vi "_crosstalk_mkpk.vi"(0 "Bias_LO_equip":T4={"Node address"=19, "CAN Interface"="CAN0", "Cartridge band"=10, "Slave Node in"={"Address"=19, "Serial Number"=[16, -88, -112, 75, 1, 8, 0, 24]}, "ObjHandle out"=93192256, "POL"=0, "sb"=1, "GPIB_SM (SIS S,V)"="24", "GPIB_DMM (SIS I)"="22", "GPIB_SM (MAG I) "="25", "GPIB_SG(LO)"="19", "GPIB_PW (PAMP) "="6", "GPIB_TMP1(8ch)"="12", "GPIB_TMP2(2ch)  "="13", "WCA_avg"=10, "Rsen"=10.0, "BiasModule"=1, "LOModule "=2, "WCA_LO_FREQ_SET"={"YTO Low freq. [GHz]"=14.66, "YTO High freq. [GHz]"=17.5, "Kvco"=1, "Lock Pol."=0, "SET LO FREQ"=88.77778, "Multiplier"=6.0, "YTO (HEX)"=197, "YTO ( FREQ)"=14.796625, "NULL PLL INTEGRATOR"=FALSE}, "Res for"=0} {"Res for" items=["none", "series res", "parallel res"]; "WCA_LO_FREQ_SET"."YTO ( FREQ)" min=25 max=150 step=0.0001 format="%.3f"; "WCA_LO_FREQ_SET"."Multiplier" min=3 max=6 step=3; "WCA_LO_FREQ_SET"."SET LO FREQ" min=25 max=150 step=0.0001 format="%.3f"; "WCA_LO_FREQ_SET"."Lock Pol." items=["Lower", "Upper"]; "WCA_LO_FREQ_SET"."Kvco" items=["7.5MHz/V", "15MHz/V"]; "WCA_LO_FREQ_SET"."YTO High freq. [GHz]" format="%.3f"; "WCA_LO_FREQ_SET"."YTO Low freq. [GHz]" format="%.3f"; "LOModule" items=["Manual Gunn+PAMP"=0, "PLL GUNN+PAMP"=5, "B10Lab LO"=1, "WCA LO"=2, ""=3, "YIG発信器"=4, "none"=99]; "BiasModule" items=["B10Lab Bias"=0, "WCA BiasModule"=1, "none"=99]; "Slave Node in"."Serial Number" format="%.0x"; "Slave Node in"."Address" format="%.0x"; "Cartridge band" max=10 step=1; "Node address" format="%.0x"}, 1 "Control":T8={"GPIB_ATT"="28", "6501Dev#"=1, "GPIB_SP"="18", "GPIB_PM"="13", "GPIB_DSA"="11", "GPIB_DMM (TPD)"="23", "GPIB_MPI"="COM9", "mortor設定"=[{"Axis"=0, "ID"=0, "HIspeed"=200.0, "LOspeed"=100.0, "ACCEL(ms)"=100.0, "Sratio"=50.0, "フリーラン\n"=FALSE, "文字列"="DSB HOT/COLD"}, {"Axis"=1, "ID"=0, "HIspeed"=4.0, "LOspeed"=4.0, "ACCEL(ms)"=100.0, "Sratio"=50.0, "フリーラン\n"=TRUE, "文字列"="SubMM Att"}, {"Axis"=0, "ID"=0, "HIspeed"=200.0, "LOspeed"=100.0, "ACCEL(ms)"=100.0, "Sratio"=50.0, "フリーラン\n"=FALSE, "文字列"="MPI Port1"}, {"Axis"=1, "ID"=0, "HIspeed"=200.0, "LOspeed"=100.0, "ACCEL(ms)"=100.0, "Sratio"=50.0, "フリーラン\n"=FALSE, "文字列"="MPI Port2"}, {"Axis"=1, "ID"=0, "HIspeed"=200.0, "LOspeed"=100.0, "ACCEL(ms)"=100.0, "Sratio"=50.0, "フリーラン\n"=TRUE, "文字列"="gainComp"}], "DATAパス"=path "C:/Documents and Settings/band10/デスクトップ/data/cartridge/CCA03/CCA-03-13/110831_etc", "mixer param file "=path "Z:/band10/Labview_ALMA/MIX95/test", "comment"="xttest", "ColdCarts"="003601", "Th"=299.0, "Tc"=77.0, "Set_SIS_volt"=2.1, "Offset"=0.0, "control"=0, "FreqLO"=799.0, "Set_Mag_Cur"=13.664233576642335, "MPI offset(mm)"=23.152, "HOT/COLD"=0} {"HOT/COLD" items=["DSB", "SBR (Cart.)", "GainComp", "SBR (MIX)"]; "control" items=["CLOSE LOOP", "OPEN LOOP", "Not Control"]}, 2 "CrossTalk_mkpk":T7={"save"=TRUE, "file_name"="xtk_799.00_120_xttest.csv", "IF start"=4.0, "IF stop"=12.0, "IF step"=1.0}, 3 "PAV配列":cluster{"VD":dbl, "VG ":dbl, "文字列":string}[](array[cluster])=[{"VD"=0.0, "VG "=-0.04, "文字列"="WCA P0"}, {"VD"=0.0, "VG "=-0.04, "文字列"="WCA P1"}, {"VD"=1.75, "VG "=2.1, "文字列"="B10 PAMP"}] {"VG" min=-1.0 max=4.0; "VD" min=0.0 max=2.5}, 4 "_LO_P_OPT":T3={"範囲配列"=[{"Start"=1.0, "Stop"=3.5, "Step"=0.01, "ｂｙ"="NEL VG"}, {"Start"=40.0, "Stop"=75.0, "Step"=1.0, "ｂｙ"="Motor"}, {"Start"=1.0, "Stop"=2.5, "Step"=0.1, "ｂｙ"="WCA VD"}], "Optimize"=0, "file_name"="LP_914.0_Tmin_100519.csv", "Save?"=FALSE, "measure"=2, "current(uA)"=60.0, "wait(ms)"=0, "IFfrq(GHz)"=8.0, "aveg"=10, "SISparam option"=2} {"SISparam option" items=["Volt and Current", "Volt only"]; "measure" items=["Pmax (only HOT)", "Tmin (HOT/COLD)", "C current"]; "Optimize" items=["Sweep", "黄金分割"]; "範囲配列"."Step" format="%.2f"; "範囲配列"."Stop" format="%.2f"; "範囲配列"."Start" format="%.2f"}) -> (7 "LOPopt P0":string="LOPt,799.00,1.46,1.88,38.10,0.00,0.00,0.00,2.10,,WCA,0.003815,4.013062,-0.021667,  1.030579,172.775269,-0.025177,")   [LabVIEW 2017]
uses:
  <vilib>/express/express arith-compare/Formula/XNode/ExpressFormulaBlockNode.xnode
panel:
  out "結果":string="4.000015,-97.540000,-93.196000,  -9.974000,-47.367000,-107.514000, -6.485000,-40.957000,-99.681000 , LOPt,799.00,1.46,1.88,38.19,0.00,0.00,0.00,2.19,,WCA,0.003662,3.952026,-0.022125,  1.031342,172.851562,-0.025787, ,LOPt,799.00,1.90,1.89,41.31,0.00,0.00,0.00,0.31,,WCA,1.335449,186.492920,-0.022125,  0.001831,3.158569,-0.025787, \n5.000041,-92.917000,-98.660000,  -10.003000,-45.366000,-102.920000, -7.055000,-44.960000,-105.715000 , LOPt,799.00,1.46,1.88,36.93,0.00,0.00,0.00,0.93,,WCA,0.003510,4.043579,-0.022736,  1.030426,172.744751,-0.025635, ,LOPt,799.00,1.90,1.90,41.12,0.00,0.00,0.00,0.12,,WCA,1.335754,186.691284,-0.021820,  0.001984,3.265381,-0.025330, \n6.000013,-94.024000,-94.568000,  -8.711000,-43.164000,-102.735000, -5.761000,-42.975000,-100.329000 , LOPt,799.00,1.46,1.87,37.45,0.00,0.00,0.00,1.45,,WCA,0.003510,3.936768,-0.022278,  1.030579,172.760010,-0.025940, ,LOPt,799.00,1.90,1.89,41.11,0.00,0.00,0.00,0.11,,WCA,1.336365,186.798096,-0.022736,  0.001831,3.173828,-0.025940, \n"
  out "XYグラフ":cluster{dbl[], dbl[]}[](graph)=[{[4.000015156, 5.000041231, 6.000013312], [-97.53999999999999, -92.917, -94.024]}, {[4.000015156, 5.000041231, 6.000013312], [-93.196, -98.66, -94.568]}]
  out "LOPopt P1":string="LOPt,799.00,1.90,1.89,41.11,0.00,0.00,0.00,0.11,,WCA,1.336365,186.798096,-0.022736,  0.001831,3.173828,-0.025940,"
  out "crossTK P1":dbl=-100.329 format="%#_6p"
  out "xpol P1":dbl=-42.975 format="%#_6p"
  out "copol P1":dbl=-5.761 format="%#_6p"
  in  "SP_set":T1={"start(GHz)"=3.5, "stop(GHz) "=12.5, "BW(MHz)"=0.0001, "VBW(Hz)"=30.0, "ref(dBm)"=0.0, "log(dB)"=15.0, "AVEG"=30, "AVEG ON/OFF"=FALSE, "Auto Align ON/OFF"=FALSE, "GPIB"="18", "point"=801}
  in  "IFBOX":T2={" Output"=1, "YIG Fc(GHz)"=4.0, " Filter"=3, "Input"=1} {"Input" items=["1:Pol 0"=1, "2:Pol 1"=2, "3:dummy"=3, "4:NoiseSource"=4]; "Filter" items=["1:YIG"=1, "2:direct"=2, "3:4-12BPF"=3, "4:direct 4-12BPF"=4]; "Output" items=["1:Speana"=1, "2:PowerMeter"=2, "3:dummy"=3, "4:TPD"=4]}
  in  "RF":T5={"RF(GHz)"=800.0, "mm_multi(4or6)"=6.0, "SGPOUT(dBm)"=10.0, "SGGPIB"="29", "PAMP GPIB"="6", "VD (V)"=1.7, "VG (V)"=2.2, "multi (V)"=8.0} {"multi (V)" min=0.0 max=15.0 step=0.5; "VG (V)" min=0.0 max=4.0 step=0.1; "VD (V)" min=0.0 max=1.85 step=0.1}
  out "crossTK P0":dbl=-102.735 format="%#_6p"
  out "xpol P0":dbl=-43.164 format="%#_6p"
  out "copol P0":dbl=-8.711 format="%#_6p"
  out "frq":dbl=6.000013312 format="%#_6p"
  in  "SIS_Deflux_heater":T6={"ON開始時間（mｓ）"=3000.0, "ON継続時間（mｓ）"=1000.0, "測定終了時間（mｓ）"=60000.0, "SIS Volt（mV)"=0.5, "GPIB_PW (SISHeater) "="3", "SAVE"=TRUE}
  out "初期時間（s）":dbl=3379641043.615625
  # "LO freq. [GHz]"
  # "YTO LOW\n/High Freq."
  # "ZERO Intgrtr"
  # "Node Address"
  # "Serial Number"
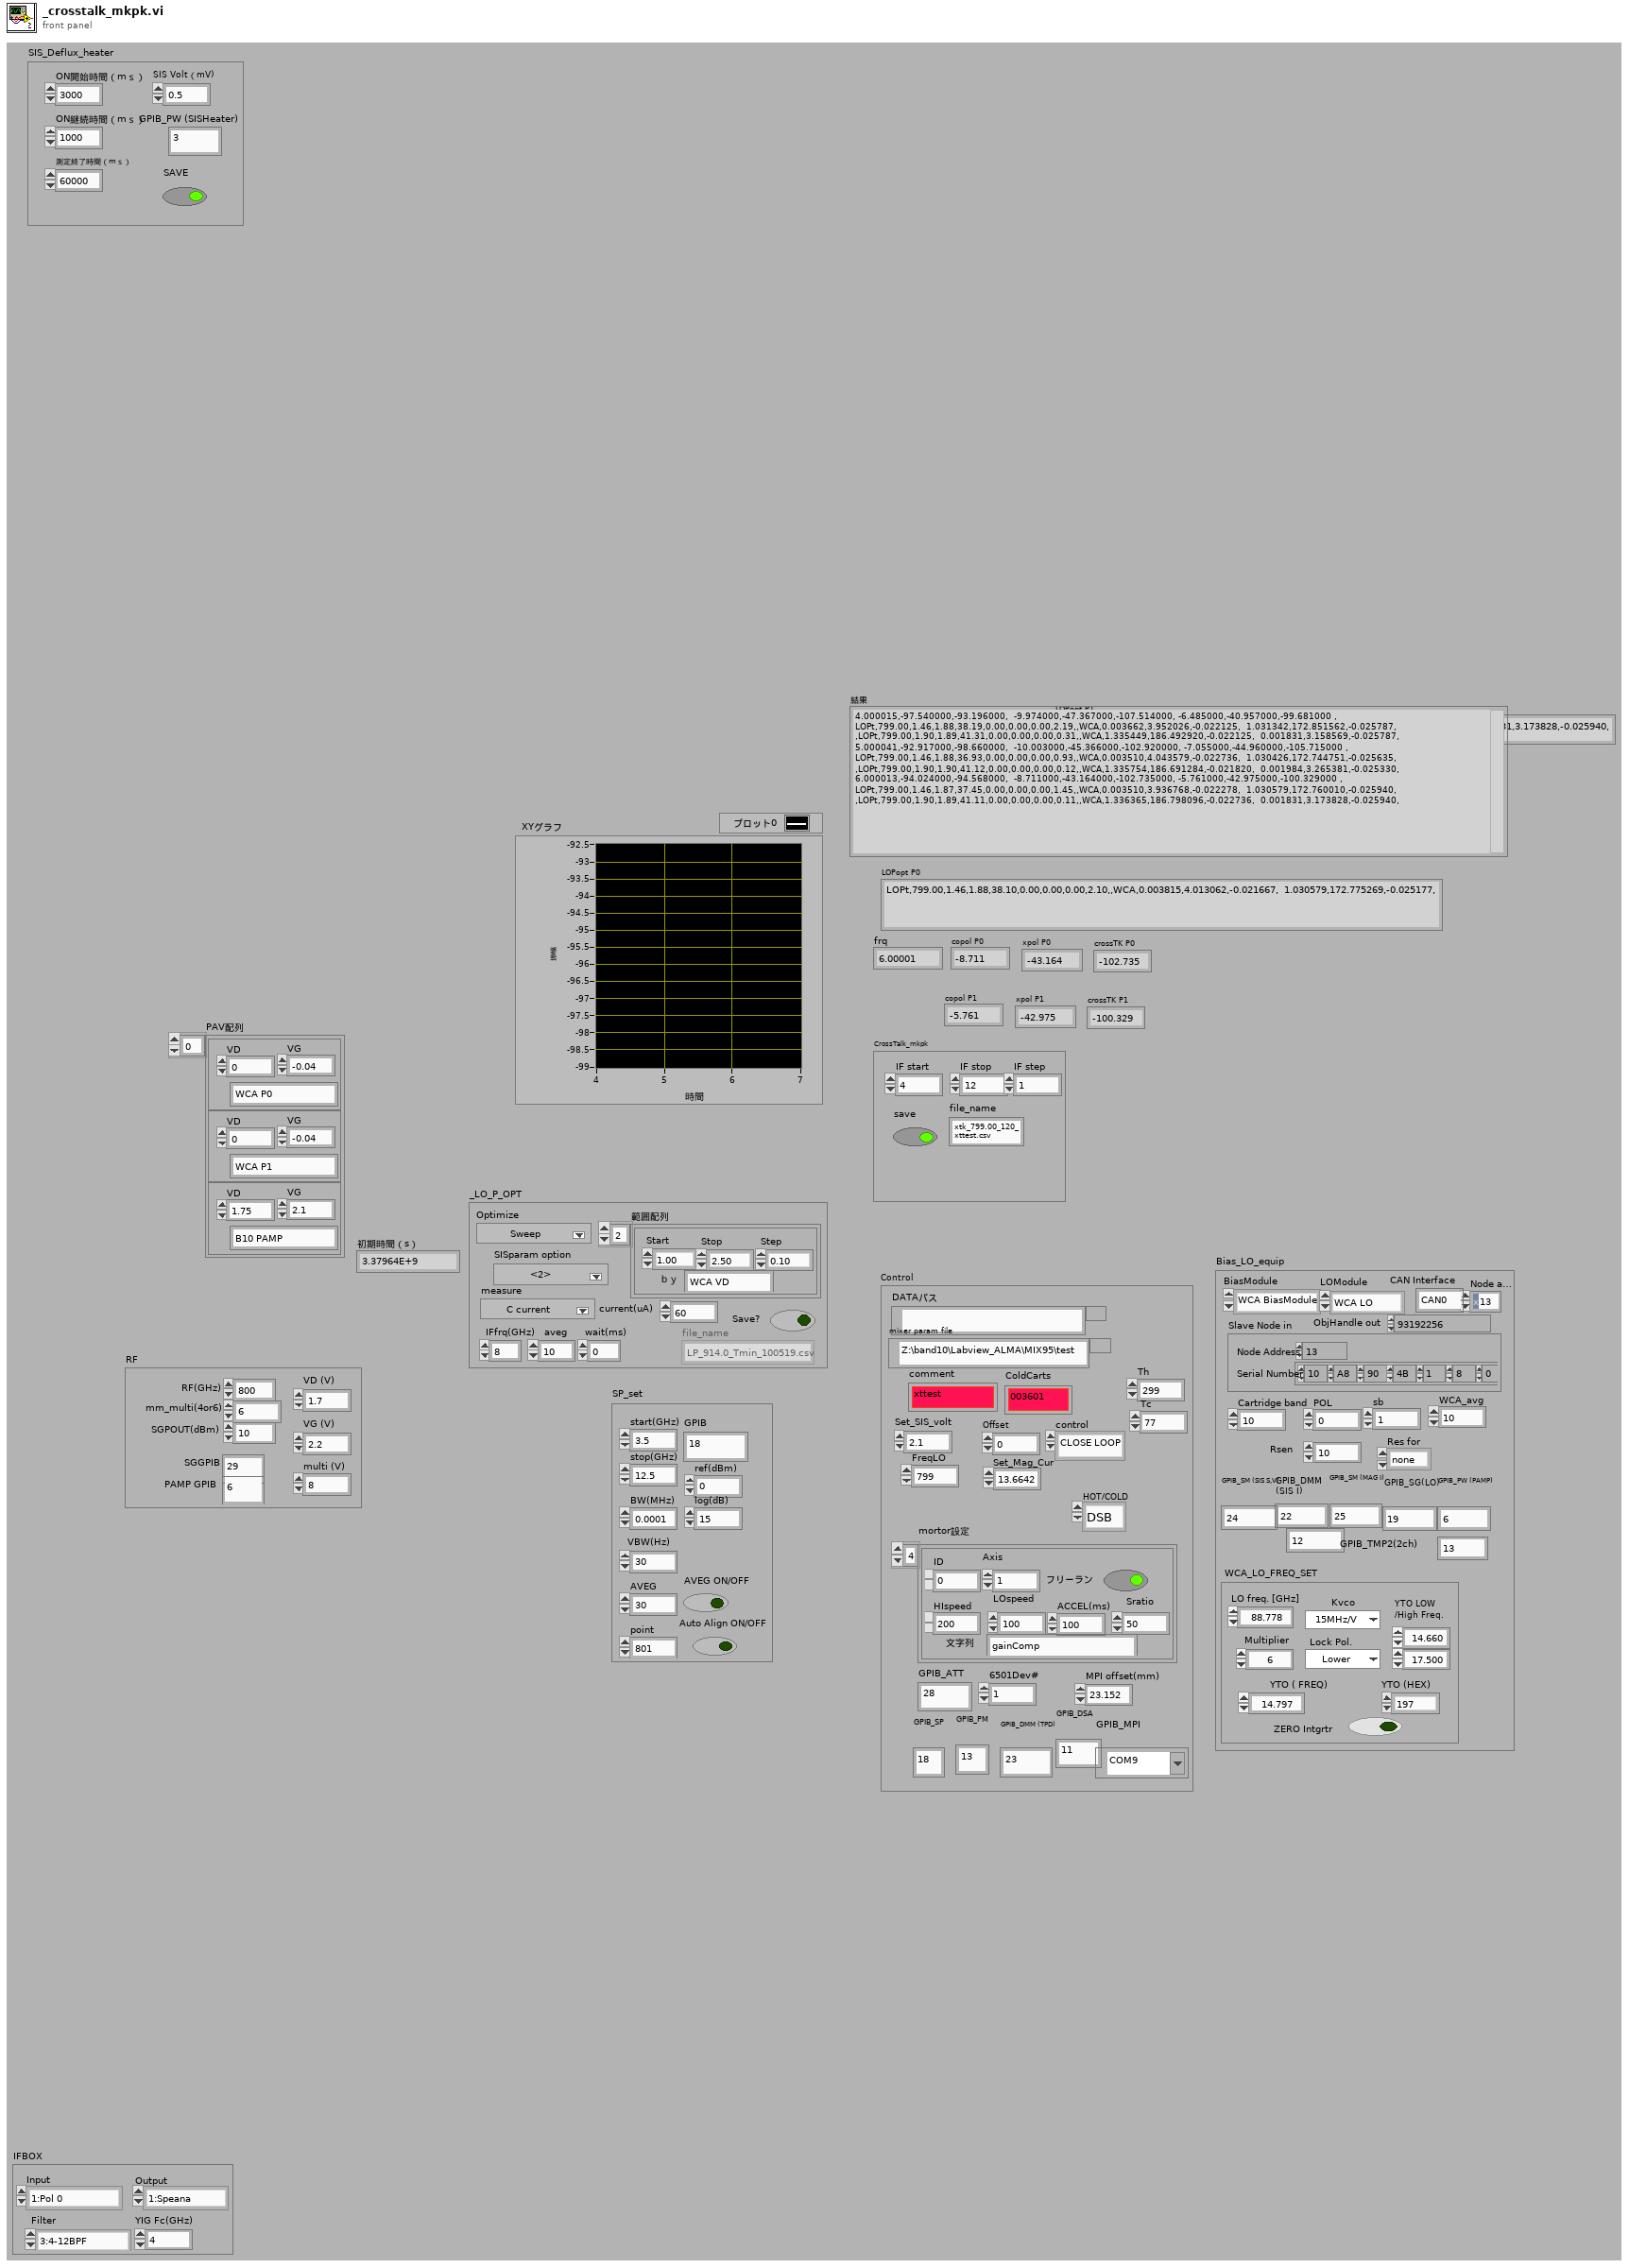
[diagram p1: front panel]
types:
  T1 = cluster{"start(GHz)":dbl, "stop(GHz) ":dbl, "BW(MHz)":dbl, "VBW(Hz)":dbl, "ref(dBm)":dbl, "log(dB)":dbl, "AVEG":i16, "AVEG ON/OFF":bool, "Auto Align ON/OFF":bool, "GPIB":string, "point":i16}
  T2 = cluster{" Output":u16, "YIG Fc(GHz)":dbl, " Filter":u16, "Input":u16}
  T3 = cluster{"範囲配列":cluster{"Start":dbl, "Stop":dbl, "Step":dbl, "ｂｙ":string}[], "Optimize":u16, "file_name":string, "Save?":bool, "measure":u16, "current(uA)":dbl, "wait(ms)":i32, "IFfrq(GHz)":dbl, "aveg":i32, "SISparam option":u16}
  T4 = cluster{"Node address":u16, "CAN Interface":string, "Cartridge band":u32, "Slave Node in":cluster{"Address":i16, "Serial Number":i8[]}, "ObjHandle out":u32, "POL":u32, "sb":u32, "GPIB_SM (SIS S,V)":string, "GPIB_DMM (SIS I)":string, "GPIB_SM (MAG I) ":string, "GPIB_SG(LO)":string, "GPIB_PW (PAMP) ":string, "GPIB_TMP1(8ch)":string, "GPIB_TMP2(2ch)  ":string, "WCA_avg":i32, "Rsen":dbl, "BiasModule":u16, "LOModule ":u16, "WCA_LO_FREQ_SET":cluster{"YTO Low freq. [GHz]":sgl, "YTO High freq. [GHz]":sgl, "Kvco":u16, "Lock Pol.":u16, "SET LO FREQ":sgl, "Multiplier":sgl, "YTO (HEX)":u16, "YTO ( FREQ)":sgl, "NULL PLL INTEGRATOR":bool}, "Res for":u16}
  T5 = cluster{"RF(GHz)":dbl, "mm_multi(4or6)":dbl, "SGPOUT(dBm)":dbl, "SGGPIB":string, "PAMP GPIB":string, "VD (V)":dbl, "VG (V)":dbl, "multi (V)":dbl}
  T6 = cluster{"ON開始時間（mｓ）":dbl, "ON継続時間（mｓ）":dbl, "測定終了時間（mｓ）":dbl, "SIS Volt（mV)":dbl, "GPIB_PW (SISHeater) ":string, "SAVE":bool}
  T7 = cluster{"save":bool, "file_name":string, "IF start":dbl, "IF stop":dbl, "IF step":dbl}
  T8 = cluster{"GPIB_ATT":string, "6501Dev#":i16, "GPIB_SP":string, "GPIB_PM":string, "GPIB_DSA":string, "GPIB_DMM (TPD)":string, "GPIB_MPI":refnum<visa-resource-name>, "mortor設定":cluster{"Axis":i16, "ID":i16, "HIspeed":dbl, "LOspeed":dbl, "ACCEL(ms)":dbl, "Sratio":dbl, "フリーラン\n":bool, "文字列":string}[], "DATAパス":path, "mixer param file ":path, "comment":string, "ColdCarts":string, "Th":dbl, "Tc":dbl, "Set_SIS_volt":dbl, "Offset":dbl, "control":u16, "FreqLO":dbl, "Set_Mag_Cur":dbl, "MPI offset(mm)":dbl, "HOT/COLD":u16}
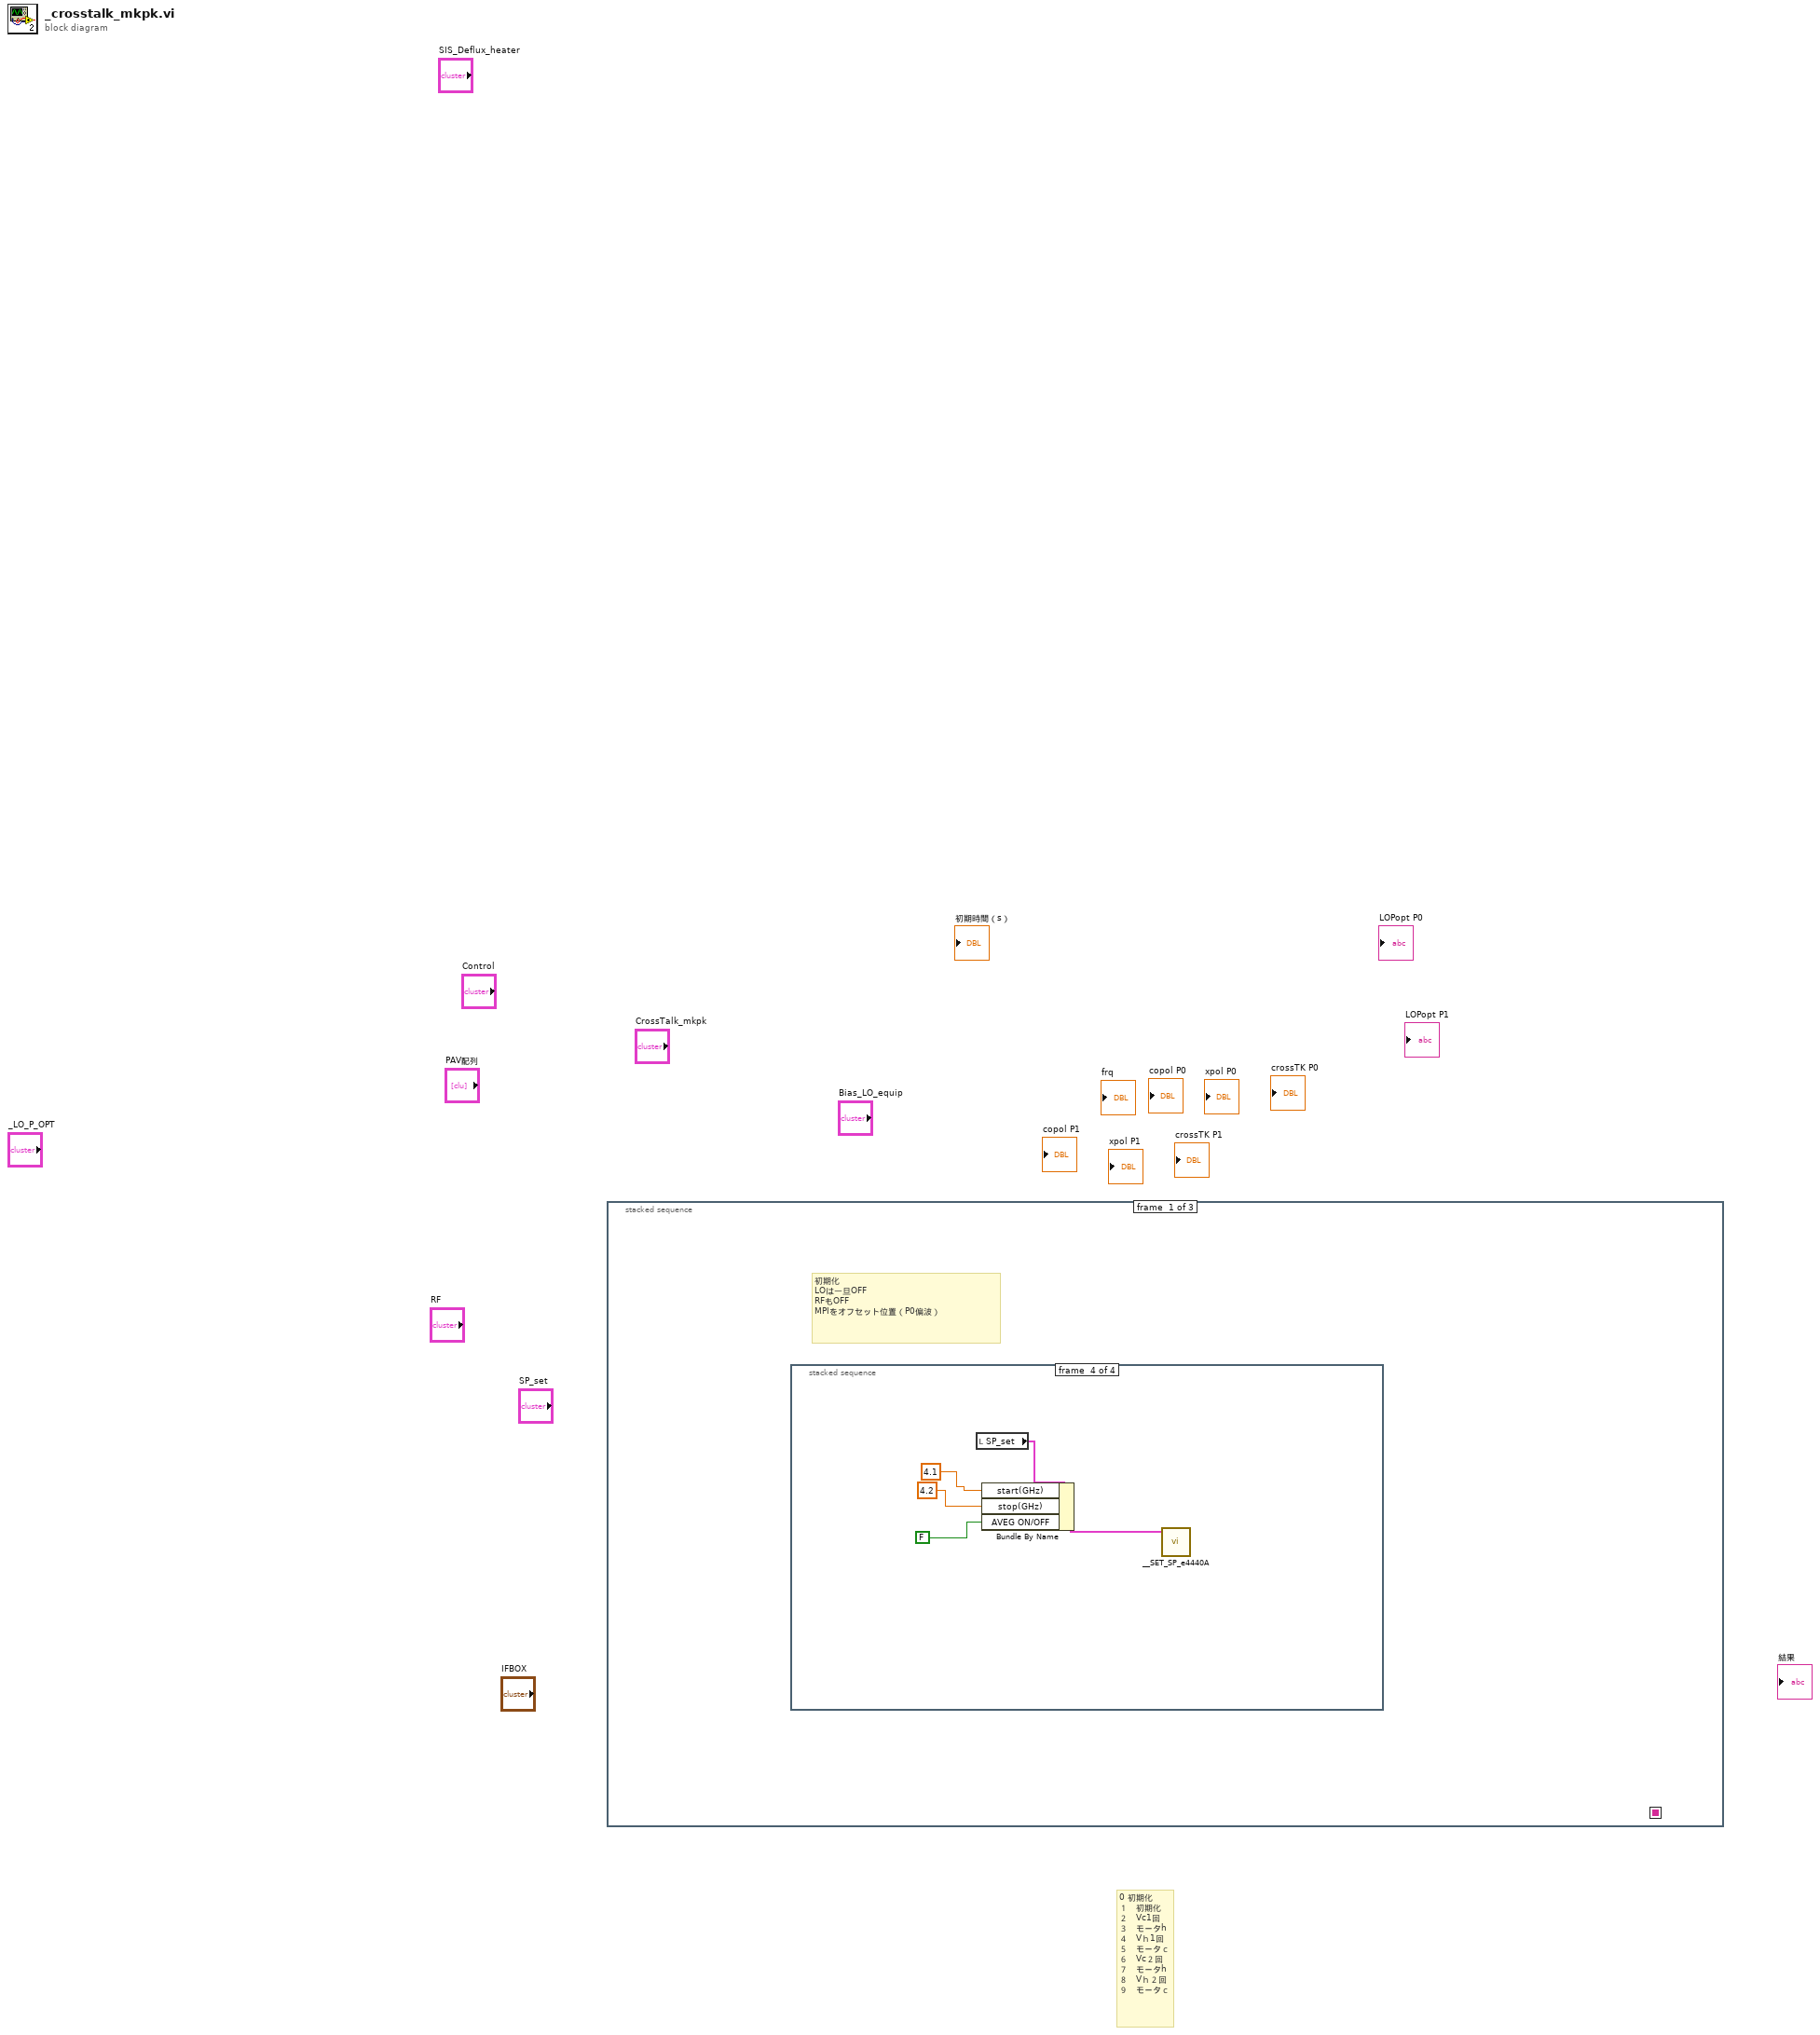
[diagram p0: block diagram]
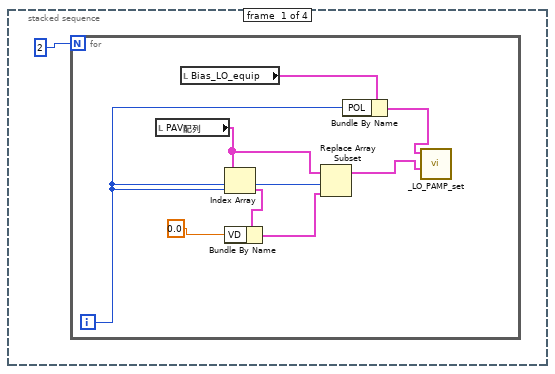
[diagram p2: hidden frame]
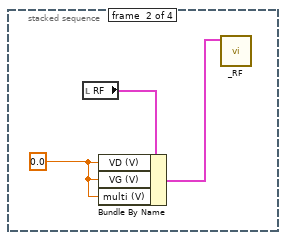
[diagram p3: hidden frame]
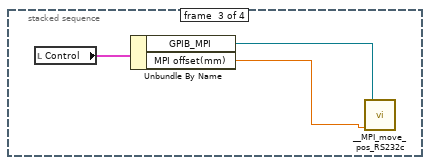
[diagram p4: hidden frame]
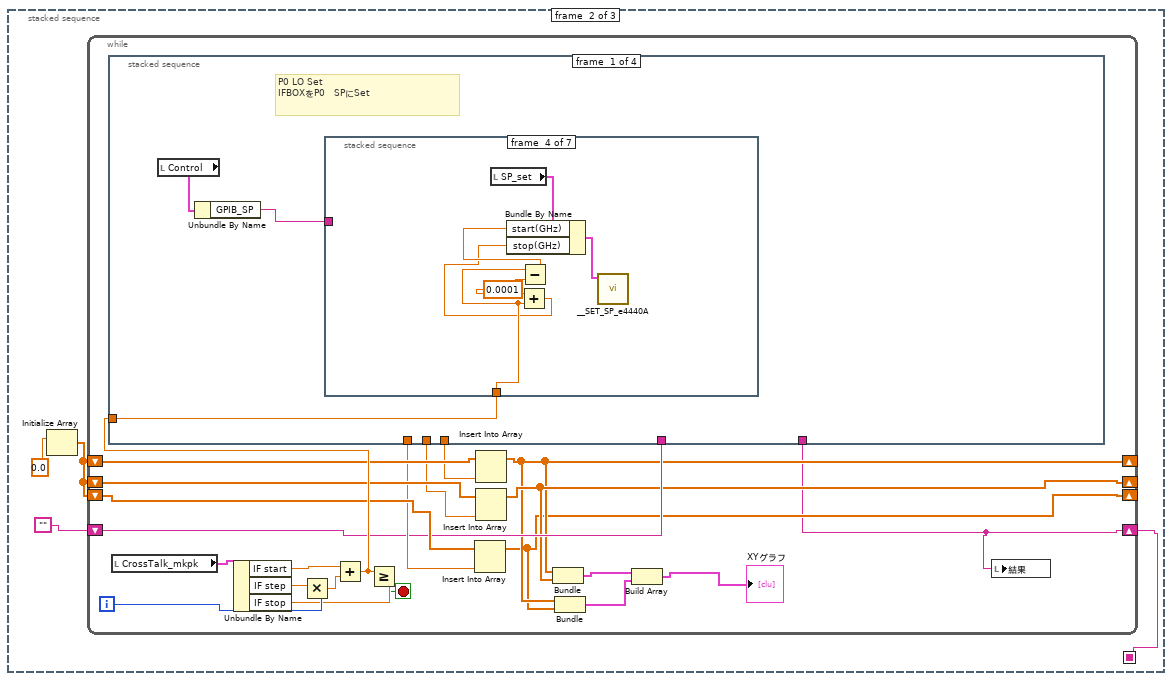
[diagram p5: hidden frame]
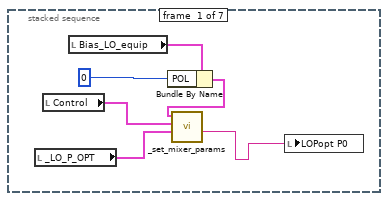
[diagram p6: hidden frame]
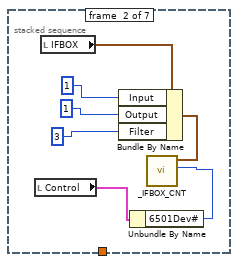
[diagram p7: hidden frame]
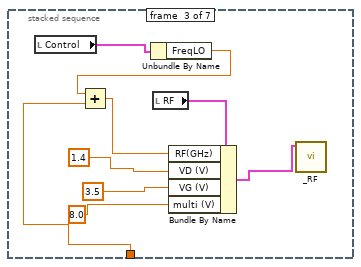
[diagram p8: hidden frame]
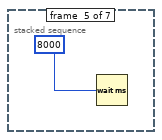
[diagram p9: hidden frame]
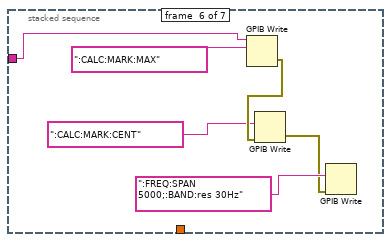
[diagram p10: hidden frame]
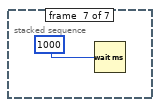
[diagram p11: hidden frame]
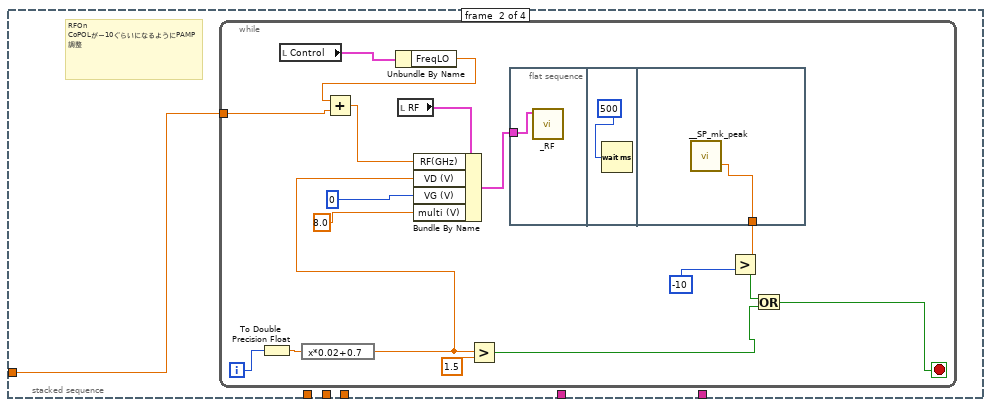
[diagram p12: hidden frame]
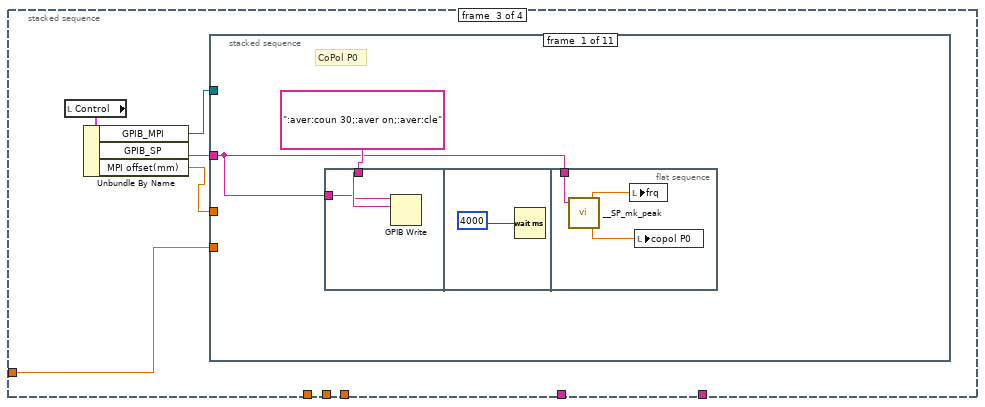
[diagram p13: hidden frame]
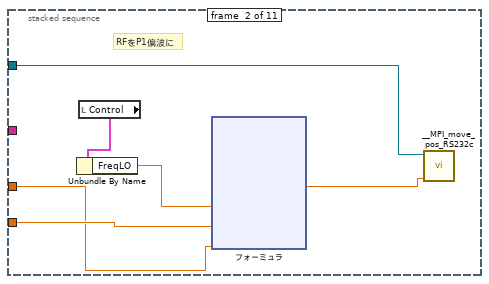
[diagram p14: hidden frame]
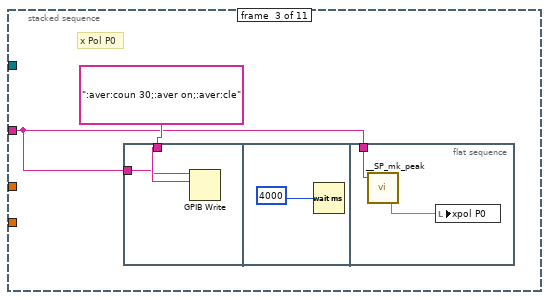
[diagram p15: hidden frame]
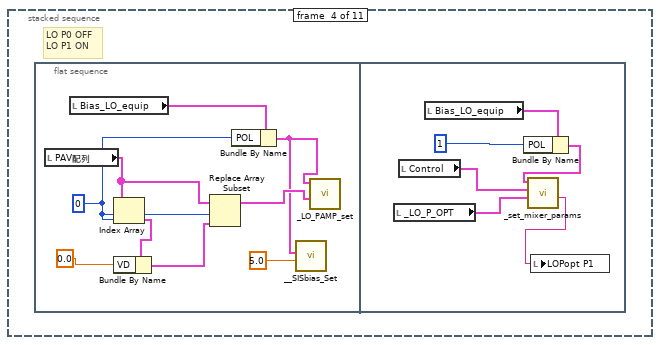
[diagram p16: hidden frame]
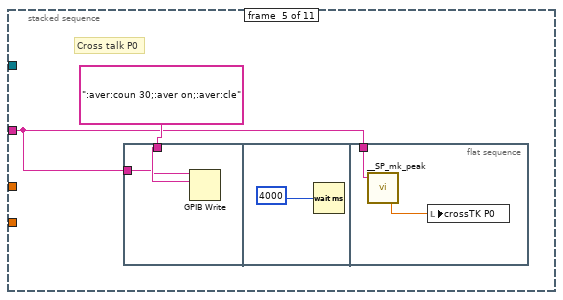
[diagram p17: hidden frame]
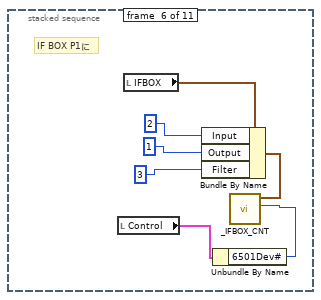
[diagram p18: hidden frame]
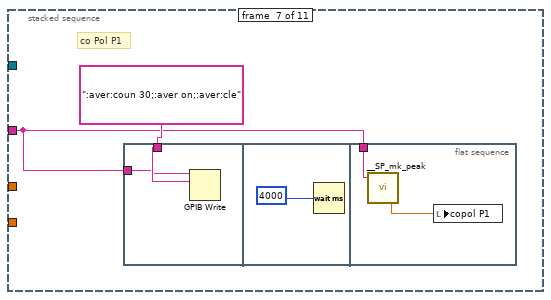
[diagram p19: hidden frame]
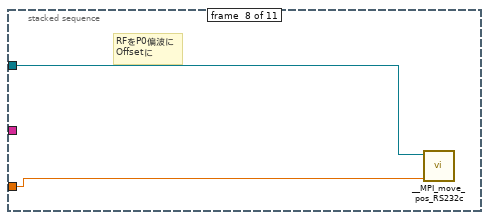
[diagram p20: hidden frame]
diagram:
  # "0 初期化\n１　初期化\n２　Vc1回\n３　モータh\n４　Vｈ1回\n５　モータｃ\n６　Vc２回\n７　モータh\n８　Vｈ２回\n９　モータｃ"
  n1 = stacked-sequence {
    seq-local: [_ w21 _] -> [_ _ w225]
    frame #0 {
      # "初期化\nLOは一旦OFF\nRFもOFF\nMPIをオフセット位置（P0偏波）"
      n2 = stacked-sequence {
        frame #0 {
          n3 = for {
            N: 2 -> [_]
            i -> [w2]
            n4 = local read "PAV配列"() -> (w5:cluster{"VD":dbl, "VG ":dbl, "文字列":string}[])
            n5 = local read "Bias_LO_equip"() -> (w4:T4)
            n6 = Index Array(array=w5, index=w2) -> (element=w8:cluster{"VD":dbl, "VG ":dbl, "文字列":string})
            n7 = Bundle By Name(cluster=w8, "VD"=0.0) -> (w9:cluster{"VD":dbl, "VG ":dbl, "文字列":string})
            n8 = Replace Array Subset(array=w5, new element=w9, index=w2) -> (w7:cluster{"VD":dbl, "VG ":dbl, "文字列":string}[])
            n9 = Bundle By Name(cluster=w4, "POL"=w2) -> (w3:T4)
            n10 = call "_LO_PAMP_set.vi"("PAV配列"=w7, "Bias_LO_equip"=w3) -> ()  [unwired: 10 in]
          }
        }
        frame #1 {
          w11 = 0.0
          n11 = local read "RF"() -> (w12:T5)
          n12 = Bundle By Name(cluster=w12, "VD (V)"=w11, "VG (V)"=w11, "multi (V)"=w11) -> (w10:T5)
          n13 = call "_RF.vi"("RF"=w10) -> ()  [unwired: 11 in]
        }
        frame #2 {
          n14 = local read "Control"() -> (w15:T8)
          n15 = Unbundle By Name(w15) -> ("GPIB_MPI"=w14:refnum<visa-resource-name>, "MPI offset(mm)"=w13:dbl)
          n16 = call "__MPI_move_pos_RS232c.vi"("pos"=w13, "VISAリソース名"=w14) -> ()  [unwired: 5 in, 1 out]
        }
        frame #3 {
          n17 = local read "SP_set"() -> (w19:T1)
          n18 = Bundle By Name(cluster=w19, "start(GHz)"=4.1, "stop(GHz)"=4.2, "AVEG ON/OFF"=FALSE) -> (w20:T1)
          n19 = call "__SET_SP_e4440A.vi"("SP"=w20) -> ()  [unwired: 7 in]
        }
      }
    }
    frame #1 {
      n20 = Initialize Array(0.0) -> (w23:dbl[])  [unwired: 1 in]
      n21 = while {
        shift-right: [w30] -> _
        shift-left: w23 -> [w38]
        shift-right: [w31] -> _
        shift-left: w23 -> [w36]
        shift-right: [w29] -> _
        shift-left: w23 -> [w34]
        shift-right: [w25] -> w21
        shift-left: "" -> [w32]
        i -> [w44]
        stop <- w40 stop-if-true
        n22 = local read "CrossTalk_mkpk"() -> (w46:T7)
        n23 = Unbundle By Name(w46) -> ("IF start"=w43:dbl, "IF step"=w45:dbl, "IF stop"=w41:dbl)
        n24 = Multiply(x=w45, y=w44) -> (x*y=w42:dbl)
        n25 = Add(x=w43, y=w42) -> (x+y=w39:dbl)
        n26 = stacked-sequence {
          tunnel: w39 -> [w49 w86 w109 _]
          tunnel: [_ _ _ w223] -> w37
          tunnel: [_ _ _ w222] -> w35
          tunnel: [_ _ _ w221] -> w33
          tunnel: w32 -> [_ _ _ w216]
          tunnel: [_ _ _ w215] -> w25
          frame #0 {
            # "P0 LO Set\nIFBOXをP0　SPにSet"
            n27 = local read "Control"() -> (w48:T8)
            n28 = Unbundle By Name(w48) -> ("GPIB_SP"=w47:string)
            n29 = stacked-sequence {
              tunnel: w49 -> [_ _ w65 w75 _ _ _]
              tunnel: w47 -> [_ _ _ _ _ w83 _]
              frame #0 {
                n30 = local read "_LO_P_OPT"() -> (w55:T3)
                n31 = local read "Control"() -> (w50:T8)
                n32 = local read "Bias_LO_equip"() -> (w54:T4)
                n33 = Bundle By Name(cluster=w54, "POL"=0) -> (w52:T4)
                n34 = call "_set_mixer_params.vi"("_LO_P_OPT"=w55, "Control"=w50, "Bias_LO_equip"=w52) -> ("文字列"=w51:string)  [unwired: 6 in, 2 out]
                n35 = local write "LOPopt P0"(w51) -> ()
              }
              frame #1 {
                n36 = local read "Control"() -> (w61:T8)
                n37 = local read "IFBOX"() -> (w60:T2)
                n38 = Bundle By Name(cluster=w60, "Input"=1, "Output"=1, "Filter"=3) -> (w59:T2)
                n39 = Unbundle By Name(w61) -> ("6501Dev#"=w62:i16)
                n40 = call "_IFBOX_CNT.vi"("6501Dev#"=w62, "IFBOX"=w59) -> ()  [unwired: 6 in]
              }
              frame #2 {
                n41 = local read "Control"() -> (w68:T8)
                n42 = Unbundle By Name(w68) -> ("FreqLO"=w66:dbl)
                n43 = Add(x=w66, y=w65) -> (x+y=w67:dbl)
                n44 = local read "RF"() -> (w71:T5)
                n45 = Bundle By Name(cluster=w71, "RF(GHz)"=w67, "VD (V)"=1.4, "VG (V)"=3.5, "multi (V)"=8.0) -> (w63:T5)
                n46 = call "_RF.vi"("RF"=w63) -> ()  [unwired: 11 in]
              }
              frame #3 {
                w74 = 0.0001
                n47 = local read "SP_set"() -> (w76:T1)
                n48 = Add(x=w74, y=w75) -> (x+y=w72:dbl)
                n49 = Subtract(x=w75, y=w74) -> (x-y=w73:dbl)
                n50 = Bundle By Name(cluster=w76, "start(GHz)"=w73, "stop(GHz)"=w72) -> (w77:T1)
                n51 = call "__SET_SP_e4440A.vi"("SP"=w77) -> ()  [unwired: 7 in]
              }
              frame #4 {
                n52 = Wait (ms)(milliseconds to wait=8000) -> ()  [unwired: 1 out]
              }
              frame #5 {
                n53 = GPIB Write(0:w83, 1:":CALC:MARK:MAX") -> (6:w82:errorcluster)  [unwired: 3 in, 1 out]
                n54 = GPIB Write(1:":CALC:MARK:CENT", 3:w82) -> (6:w79:errorcluster)  [unwired: 3 in, 1 out]
                n55 = GPIB Write(1:":FREQ:SPAN 5000;:BAND:res 30Hz", 3:w79) -> ()  [unwired: 3 in, 2 out]
              }
              frame #6 {
                n56 = Wait (ms)(milliseconds to wait=1000) -> ()  [unwired: 1 out]
              }
            }
          }
          frame #1 {
            # "RFOn\nCoPOLがー10ぐらいになるようにPAMP調整"
            n57 = while {
              tunnel: w86 -> [w87]
              i -> [w103]
              stop <- w91 stop-if-true
              n58 = To Double Precision Float(number=w103) -> (double precision float=w102:dbl)
              n59 = local read "Control"() -> (w90:T8)
              n60 = expression code="x*0.02+0.7"(w102) -> (w98:dbl)
              n61 = Unbundle By Name(w90) -> ("FreqLO"=w88:dbl)
              n62 = Add(x=w88, y=w87) -> (x+y=w89:dbl)
              n63 = local read "RF"() -> (w100:T5)
              n64 = Bundle By Name(cluster=w100, "RF(GHz)"=w89, "VD (V)"=w98, "VG (V)"=0, "multi (V)"=8.0) -> (w99:T5)
              n65 = Greater?(x=w98, y=1.5) -> (0:w92:bool)
              n66 = flat-sequence {
                tunnel: w99 -> [w104]
                tunnel: [w106] -> w95
                frame #0 {
                  n67 = call "_RF.vi"("RF"=w104) -> ()  [unwired: 11 in]
                }
                frame #1 {
                  n68 = Wait (ms)(milliseconds to wait=500) -> ()  [unwired: 1 out]
                }
                frame #2 {
                  n69 = call "__SP_mk_peak.vi"() -> ("pow out"=w106:dbl)  [unwired: 3 in, 1 out]
                }
              }
              n70 = Greater?(x=w95, y=-10) -> (0:w93:bool)
              n71 = Or(x=w93, y=w92) -> (x .or. y?=w91:bool)
            }
          }
          frame #2 {
            n72 = local read "Control"() -> (w111:T8)
            n73 = Unbundle By Name(w111) -> ("GPIB_MPI"=w107:refnum<visa-resource-name>, "GPIB_SP"=w110:string, "MPI offset(mm)"=w108:dbl)
            n74 = stacked-sequence {
              tunnel: w110 -> [w112 _ w138 _ w160 _ w174 _ w183 _ w204]
              tunnel: w109 -> [_ w123 _ _ _ _ _ _ _ _ _]
              tunnel: w108 -> [_ w122 _ _ _ _ _ w181 _ _ _]
              tunnel: w107 -> [_ w121 _ _ _ _ _ w182 _ _ _]
              frame #0 {
                # "CoPol P0"
                n75 = flat-sequence {
                  tunnel: ":aver:coun 30;:aver on;:aver:cle" -> [w115]
                  tunnel: w112 -> [w114]
                  tunnel: w112 -> [w117]
                  frame #0 {
                    n76 = GPIB Write(0:w114, 1:w115) -> ()  [unwired: 3 in, 2 out]
                  }
                  frame #1 {
                    n77 = Wait (ms)(milliseconds to wait=4000) -> ()  [unwired: 1 out]
                  }
                  frame #2 {
                    n78 = call "__SP_mk_peak.vi"("GIPB番号"=w117) -> ("pow out"=w118:dbl, "Freq out"=w119:dbl)  [unwired: 2 in]
                    n79 = local write "frq"(w119) -> ()
                    n80 = local write "copol P0"(w118) -> ()
                  }
                }
              }
              frame #1 {
                # "RFをP1偏波に"
                n81 = local read "Control"() -> (w125:T8)
                n82 = Unbundle By Name(w125) -> ("FreqLO"=w124:dbl)
                n83 = xnode "フォーミュラ"("LO"=w124, "IF"=w123, "offset"=w122) -> ("結果"=w120:dbl)  [unwired: 1 in, 1 out]
                n84 = call "__MPI_move_pos_RS232c.vi"("pos"=w120, "VISAリソース名"=w121) -> ()  [unwired: 5 in, 1 out]
              }
              frame #2 {
                # "x Pol P0"
                n85 = flat-sequence {
                  tunnel: ":aver:coun 30;:aver on;:aver:cle" -> [w141]
                  tunnel: w138 -> [w140]
                  tunnel: w138 -> [w143]
                  frame #0 {
                    n86 = GPIB Write(0:w140, 1:w141) -> ()  [unwired: 3 in, 2 out]
                  }
                  frame #1 {
                    n87 = Wait (ms)(milliseconds to wait=4000) -> ()  [unwired: 1 out]
                  }
                  frame #2 {
                    n88 = call "__SP_mk_peak.vi"("GIPB番号"=w143) -> ("pow out"=w144:dbl)  [unwired: 2 in, 1 out]
                    n89 = local write "xpol P0"(w144) -> ()
                  }
                }
              }
              frame #3 {
                # "LO P0 OFF\nLO P1 ON"
                n90 = flat-sequence {
                  frame #0 {
                    w147 = 0
                    n91 = local read "PAV配列"() -> (w149:cluster{"VD":dbl, "VG ":dbl, "文字列":string}[])
                    n92 = local read "Bias_LO_equip"() -> (w148:T4)
                    n93 = Index Array(array=w149, index=w147) -> (element=w152:cluster{"VD":dbl, "VG ":dbl, "文字列":string})
                    n94 = Bundle By Name(cluster=w152, "VD"=0.0) -> (w153:cluster{"VD":dbl, "VG ":dbl, "文字列":string})
                    n95 = Replace Array Subset(array=w149, new element=w153, index=w147) -> (w151:cluster{"VD":dbl, "VG ":dbl, "文字列":string}[])
                    n96 = Bundle By Name(cluster=w148, "POL"=w147) -> (w146:T4)
                    n97 = call "__SISbias_Set.vi"("Set_V"=5.0, "Bias_LO_equip"=w146) -> ()  [unwired: 9 in, 1 out]
                    n98 = call "_LO_PAMP_set.vi"("PAV配列"=w151, "Bias_LO_equip"=w146) -> ()  [unwired: 10 in]
                  }
                  frame #1 {
                    n99 = local read "_LO_P_OPT"() -> (w159:T3)
                    n100 = local read "Control"() -> (w154:T8)
                    n101 = local read "Bias_LO_equip"() -> (w158:T4)
                    n102 = Bundle By Name(cluster=w158, "POL"=1) -> (w156:T4)
                    n103 = call "_set_mixer_params.vi"("_LO_P_OPT"=w159, "Control"=w154, "Bias_LO_equip"=w156) -> ("文字列"=w155:string)  [unwired: 6 in, 2 out]
                    n104 = local write "LOPopt P1"(w155) -> ()
                  }
                }
              }
              frame #4 {
                # "Cross talk P0"
                n105 = flat-sequence {
                  tunnel: ":aver:coun 30;:aver on;:aver:cle" -> [w163]
                  tunnel: w160 -> [w162]
                  tunnel: w160 -> [w165]
                  frame #0 {
                    n106 = GPIB Write(0:w162, 1:w163) -> ()  [unwired: 3 in, 2 out]
                  }
                  frame #1 {
                    n107 = Wait (ms)(milliseconds to wait=4000) -> ()  [unwired: 1 out]
                  }
                  frame #2 {
                    n108 = call "__SP_mk_peak.vi"("GIPB番号"=w165) -> ("pow out"=w166:dbl)  [unwired: 2 in, 1 out]
                    n109 = local write "crossTK P0"(w166) -> ()
                  }
                }
              }
              frame #5 {
                # "IF BOX P1に"
                n110 = local read "Control"() -> (w172:T8)
                n111 = local read "IFBOX"() -> (w171:T2)
                n112 = Bundle By Name(cluster=w171, "Input"=2, "Output"=1, "Filter"=3) -> (w170:T2)
                n113 = Unbundle By Name(w172) -> ("6501Dev#"=w173:i16)
                n114 = call "_IFBOX_CNT.vi"("6501Dev#"=w173, "IFBOX"=w170) -> ()  [unwired: 6 in]
              }
              frame #6 {
                # "co Pol P1"
                n115 = flat-sequence {
                  tunnel: ":aver:coun 30;:aver on;:aver:cle" -> [w177]
                  tunnel: w174 -> [w176]
                  tunnel: w174 -> [w179]
                  frame #0 {
                    n116 = GPIB Write(0:w176, 1:w177) -> ()  [unwired: 3 in, 2 out]
                  }
                  frame #1 {
                    n117 = Wait (ms)(milliseconds to wait=4000) -> ()  [unwired: 1 out]
                  }
                  frame #2 {
                    n118 = call "__SP_mk_peak.vi"("GIPB番号"=w179) -> ("pow out"=w180:dbl)  [unwired: 2 in, 1 out]
                    n119 = local write "copol P1"(w180) -> ()
                  }
                }
              }
              frame #7 {
                # "RFをP0偏波に\nOffsetに"
                n120 = call "__MPI_move_pos_RS232c.vi"("pos"=w181, "VISAリソース名"=w182) -> ()  [unwired: 5 in, 1 out]
              }
              frame #8 {
                # "X Pol P1"
                n121 = flat-sequence {
                  tunnel: ":aver:coun 30;:aver on;:aver:cle" -> [w186]
                  tunnel: w183 -> [w185]
                  tunnel: w183 -> [w188]
                  frame #0 {
                    n122 = GPIB Write(0:w185, 1:w186) -> ()  [unwired: 3 in, 2 out]
                  }
                  frame #1 {
                    n123 = Wait (ms)(milliseconds to wait=4000) -> ()  [unwired: 1 out]
                  }
                  frame #2 {
                    n124 = call "__SP_mk_peak.vi"("GIPB番号"=w188) -> ("pow out"=w189:dbl)  [unwired: 2 in, 1 out]
                    n125 = local write "xpol P1"(w189) -> ()
                  }
                }
              }
              frame #9 {
                # "LO P1 OFF\nLO P０ ON"
                n126 = flat-sequence {
                  frame #0 {
                    w192 = 1
                    n127 = local read "PAV配列"() -> (w194:cluster{"VD":dbl, "VG ":dbl, "文字列":string}[])
                    n128 = local read "Bias_LO_equip"() -> (w193:T4)
                    n129 = Index Array(array=w194, index=w192) -> (element=w197:cluster{"VD":dbl, "VG ":dbl, "文字列":string})
                    n130 = Bundle By Name(cluster=w197, "VD"=0.0) -> (w198:cluster{"VD":dbl, "VG ":dbl, "文字列":string})
                    n131 = Replace Array Subset(array=w194, new element=w198, index=w192) -> (w196:cluster{"VD":dbl, "VG ":dbl, "文字列":string}[])
                    n132 = Bundle By Name(cluster=w193, "POL"=w192) -> (w190:T4)
                    n133 = call "__SISbias_Set.vi"("Set_V"=5.0, "Bias_LO_equip"=w190) -> ()  [unwired: 9 in, 1 out]
                    n134 = call "_LO_PAMP_set.vi"("PAV配列"=w196, "Bias_LO_equip"=w190) -> ()  [unwired: 10 in]
                  }
                  frame #1 {
                    n135 = local read "_LO_P_OPT"() -> (w203:T3)
                    n136 = local read "Control"() -> (w199:T8)
                    n137 = local read "Bias_LO_equip"() -> (w202:T4)
                    n138 = Bundle By Name(cluster=w202, "POL"=0) -> (w200:T4)
                    n139 = call "_set_mixer_params.vi"("_LO_P_OPT"=w203, "Control"=w199, "Bias_LO_equip"=w200) -> ()  [unwired: 6 in, 3 out]
                  }
                }
              }
              frame #10 {
                # "cross talk P1"
                n140 = flat-sequence {
                  tunnel: ":aver:coun 30;:aver on;:aver:cle" -> [w207]
                  tunnel: w204 -> [w206]
                  tunnel: w204 -> [w209]
                  frame #0 {
                    n141 = GPIB Write(0:w206, 1:w207) -> ()  [unwired: 3 in, 2 out]
                  }
                  frame #1 {
                    n142 = Wait (ms)(milliseconds to wait=4000) -> ()  [unwired: 1 out]
                  }
                  frame #2 {
                    n143 = call "__SP_mk_peak.vi"("GIPB番号"=w209) -> ("pow out"=w210:dbl)  [unwired: 2 in, 1 out]
                    n144 = local write "crossTK P1"(w210) -> ()
                  }
                }
              }
            }
          }
          frame #3 {
            n145 = local read "xpol P0"() -> (w220:dbl)
            n146 = local read "crossTK P0"() -> (w213:dbl)
            n147 = local read "crossTK P1"() -> (w211:dbl)
            n148 = local read "copol P0"() -> (w214:dbl)
            n149 = local read "copol P1"() -> (w212:dbl)
            n150 = local read "xpol P1"() -> (w219:dbl)
            n151 = local read "frq"() -> (w223:dbl)
            n152 = Subtract(x=w211, y=w212) -> (x-y=w221:dbl)
            n153 = Subtract(x=w213, y=w214) -> (x-y=w222:dbl)
            n154 = local read "LOPopt P0"() -> (w218:string)
            n155 = local read "LOPopt P1"() -> (w217:string)
            n156 = Format Into String(format string="%f,%f,%f,  %f,%f,%f, %f,%f,%f , %s ,%s \\n", initial string=w216, w223, w222, w221, w214, w220, w213, w212, w219, w211, w218, w217) -> (resulting string=w215:string)  [unwired: 1 in, 1 out]
          }
        }
        n157 = Greater Or Equal?(x=w39, y=w41) -> (x >= y?=w40:bool)
        n158 = Insert Into Array(array=w34, new element=w33) -> (w29:dbl[])  [unwired: 1 in]
        n159 = Insert Into Array(array=w38, new element=w37) -> (w30:dbl[])  [unwired: 1 in]
        n160 = Insert Into Array(array=w36, new element=w35) -> (w31:dbl[])  [unwired: 1 in]
        n161 = Bundle(w30, w31) -> (w28:cluster{dbl[], dbl[]})  [unwired: 1 in]
        n162 = Bundle(w30, w29) -> (w27:cluster{dbl[], dbl[]})  [unwired: 1 in]
        n163 = Build Array(w28, w27) -> (→"XYグラフ":cluster{dbl[], dbl[]}[])
        n164 = local write "結果"(w25) -> ()
      }
    }
    frame #2 {
      n165 = local read "CrossTalk_mkpk"() -> (w230:T7)
      n166 = local read "Control"() -> (w227:T8)
      n167 = Unbundle By Name(w227) -> ("DATAパス"=w226:path)
      n168 = Unbundle By Name(w230) -> ("save"=w229:bool, "file_name"=w228:string)
      n169 = case shown="참" w229 {
        tunnel: w228 -> [_ w235]
        tunnel: w226 -> [_ w234]
        tunnel: w225 -> [_ w231]
        frame False {
        }
        frame True {
          n170 = Equal?(x=w234, y=path "") -> (x = y?=w236:bool)
          n171 = String Length(string=w235) -> (length=w241:i32)
          n172 = Equal?(x=w241, y=0) -> (x = y?=w237:bool)
          n173 = Or(x=w237, y=w236) -> (x .or. y?=w238:bool)
          n174 = case shown="참" w238 {
            tunnel: w235 -> [w250 _]
            tunnel: [w249 w252] -> w233
            tunnel: [FALSE w251] -> w232
            tunnel: w234 -> [w247 _]
            frame False {
              n175 = Build Path(base path=w247, name or relative path=w250) -> (appended path=w249:path)
            }
            frame True {
              n176 = Open/Create/Replace File(operation (0:open)=5) -> (refnum out=w253:refnum<file>, cancelled=w251:bool)  [unwired: 5 in, 1 out]
              n177 = case shown="거짓" w251 {
                tunnel: w253 -> [w256 _]
                tunnel: [w255 path ""] -> w252
                frame False {
                  n178 = Close File(refnum=w256) -> (path=w255:path)  [unwired: 1 in, 1 out]
                }
                frame True {
                }
              }
            }
          }
          n179 = case shown="참" w232 {
            tunnel: w233 -> [w246 _]
            tunnel: w231 -> [w242 _]
            frame False {
              n180 = Open/Create/Replace File(file path (use dialog)=w246, operation (0:open)=4) -> (refnum out=w244:refnum<file>)  [unwired: 4 in, 2 out]
              n181 = Write to Text File(file (use dialog)=w244, text=w242) -> (refnum out=w243:refnum<file>)  [unwired: 2 in, 2 out]
              n182 = Close File(refnum=w243) -> ()  [unwired: 1 in, 2 out]
            }
            frame True {
            }
          }
        }
      }
    }
  }
